vi "initialize.vi"(8 "error in (no error)":errorcluster, 11 "PI_Piezo in":refnum<class "PI_Piezo.lvclass">) -> (0 "error out":errorcluster, 3 "PI_Piezo out":refnum<class "PI_Piezo.lvclass">)   [LabVIEW 2013, in "PI_Piezo.lvclass"]
uses:
  PI_Piezo.lvclass
  PI_Piezo.lvclass/PI_Piezo.ctl
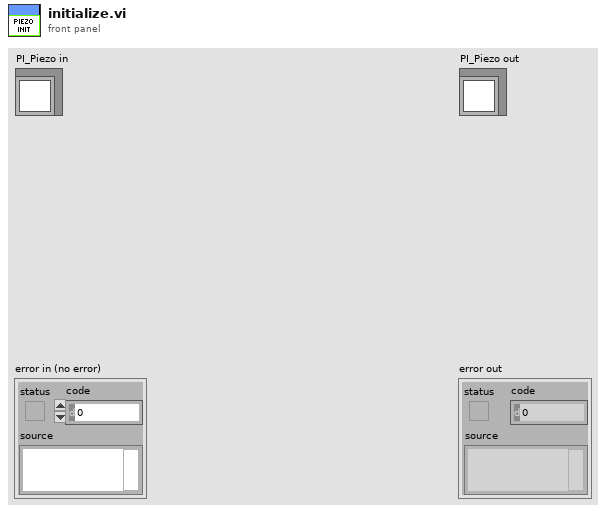
[diagram p1: front panel]
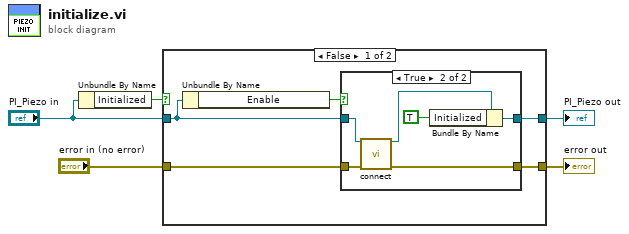
[diagram p0: block diagram]
diagram:
  n1 = Unbundle By Name("PI_Piezo in") -> ("Initialized"=w2:bool)
  n2 = case shown="False" w2 {
    tunnel: [w6 w19] -> w5
    tunnel: [w8 w20] -> w4
    tunnel: "PI_Piezo in" -> [w9 w20]
    tunnel: "error in (no error)" -> [w7 w19]
    frame False {
      n3 = Unbundle By Name(w9) -> ("Enable"=w10:bool)
      n4 = case shown="True" w10 {
        tunnel: w9 -> [w11 w18]
        tunnel: [w11 w14] -> w8
        tunnel: w7 -> [w12 w17]
        tunnel: [w12 w16] -> w6
        frame False {
        }
        frame True {
          n5 = call "connect.vi"("PI_Piezo.lvclass (in)"=w18, "error in"=w17) -> ("PI_Piezo.lvclass"=w15:refnum<class "PI_Piezo.lvclass">, "error out"=w16:errorcluster)  [unwired: 12 in]
          n6 = Bundle By Name(cluster=w15, "Initialized"=TRUE) -> (w14:refnum<class "PI_Piezo.lvclass">)
        }
      }
    }
    frame True {
    }
  }
  "error out" <- w5
  "PI_Piezo out" <- w4
